vi "executeTask.vi"(7 "VisibleTask?":bool, 8 "error in (no error)":errorcluster, 9 "Parameters":variant, 10 "Task":string, 11 "pdbm_testsys_reqst_event":refnum<user-event>) -> (0 "error IO":errorcluster, 3 "pdbm_testsys_reqst_event out":refnum<user-event>)   [LabVIEW 2015, in "pdbm_test_system.lvlib"]
doc: "call VI specified by its name."
uses:
  pdbm_test_system.lvlib
  pdbm_testsys_taskroute_inter/UsrDefine/pdbm_testsys_reqst_data.ctl
  pdbm_testsys_taskroute_inter/pdbm_testsys_taskroute_inter.lvlib
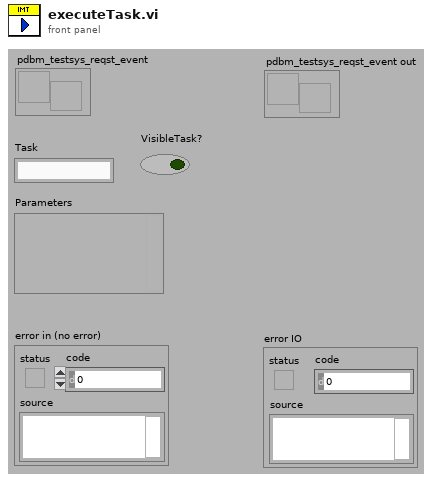
[diagram p1: front panel]
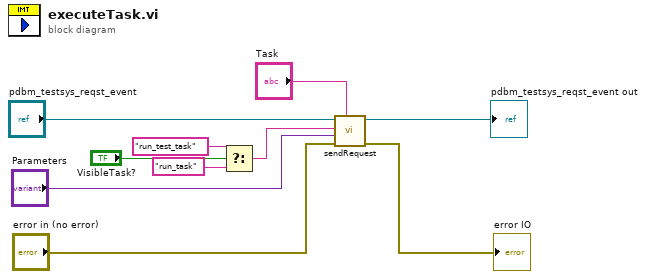
[diagram p0: block diagram]
diagram:
  n1 = Select(t="run_test_task", s="VisibleTask?", f="run_task" ("Request")) -> (s? t:f=w1:string)
  n2 = call "sendRequest.vi"("TaskName"="Task", "error in (no error)"="error in (no error)", "Parameters"="Parameters", "Request"=w1, "pdbm_testsys_reqst_event"="pdbm_testsys_reqst_event") -> ("error IO"=→"error IO":errorcluster, "pdbm_testsys_reqst_event out"=→"pdbm_testsys_reqst_event out":refnum<user-event>)  [unwired: 5 in]
